vi "Merge Driver Call by Reference Error.vi"(8 "driver name":string, 10 "called vi error":errorcluster, 11 "call by ref error":errorcluster) -> (2 "error out":errorcluster)   [LabVIEW 2020, in "NI Session Management Instrument.lvlib" / "ISession Factory.lvclass"]
uses:
  ISession Factory.lvclass
  Measurements/Helpers/Error Strings Global Internal.vi
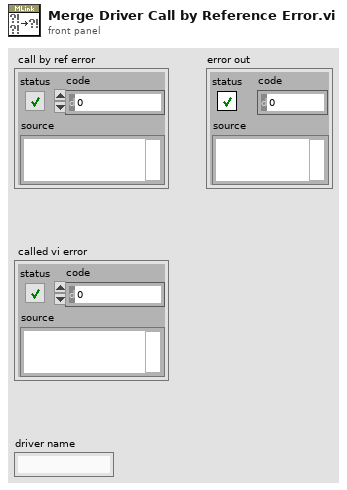
[diagram p1: front panel]
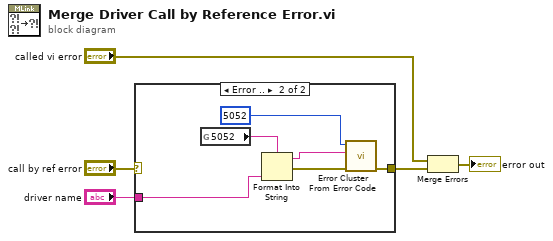
[diagram p0: block diagram]
diagram:
  n1 = case shown="Error .." "call by ref error" {
    selector: "call by ref error" -> [w6 _]
    tunnel: [w6 w8] -> w3
    tunnel: "driver name" -> [_ w7]
    frame No Error {
    }
    frame Error {
      n2 = global read "Error Strings Global Internal.vi" "5052"() -> (w10:string)
      n3 = Format Into String(format string=w10, w7) -> (resulting string=w11:string, error out=w12:errorcluster)  [unwired: 2 in]
      n4 = call <vilib>:"Error Cluster From Error Code.vi"("error in (no error)"=w12, "error message (\"\")"=w11, "error code (0)"=5052) -> ("error out"=w8:errorcluster)  [unwired: 6 in]
    }
  }
  n5 = Merge Errors("called vi error", w3) -> (→"error out":errorcluster)
